vi "Tranzycja.vi"(7 "input":T2, 9 "Tranzycja":bool, 11 "Interlock":bool) -> (3 "Akcja":bool, 4 "output":T2)   [LabVIEW 2020]
uses:
  controls/Data.ctl
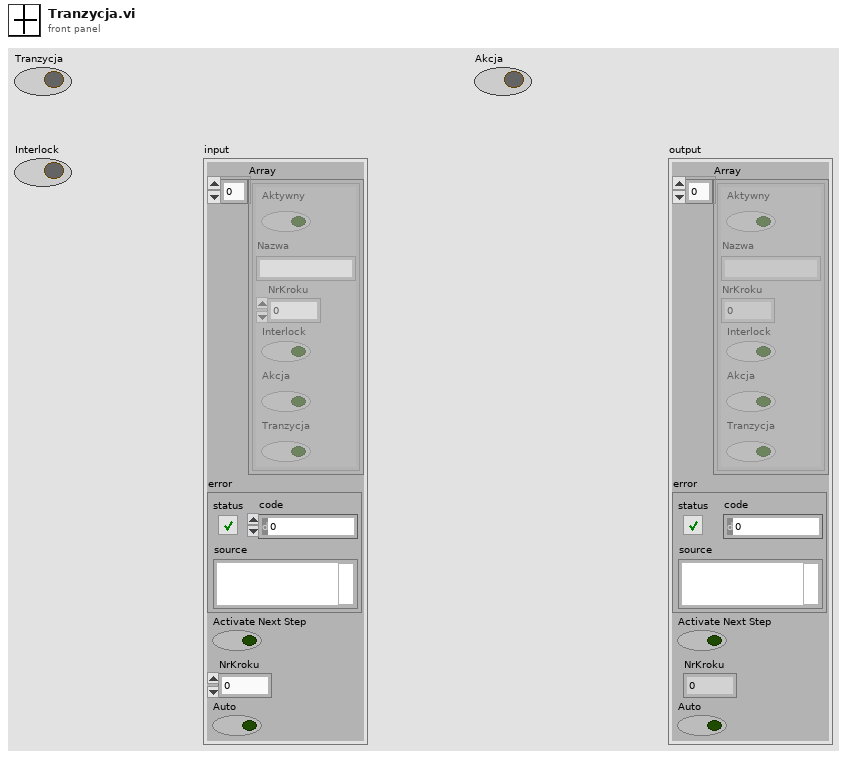
[diagram p1: front panel]
types:
  T1 = typedef "Data.ctl" = cluster{"Aktywny":bool, "Nazwa":string, "NrKroku":dbl, "Interlock":bool, "Akcja":bool, "Tranzycja":bool}
  T2 = cluster{"Array":T1[], "error":errorcluster, "Activate Next Step":bool, "NrKroku":dbl, "Auto":bool}
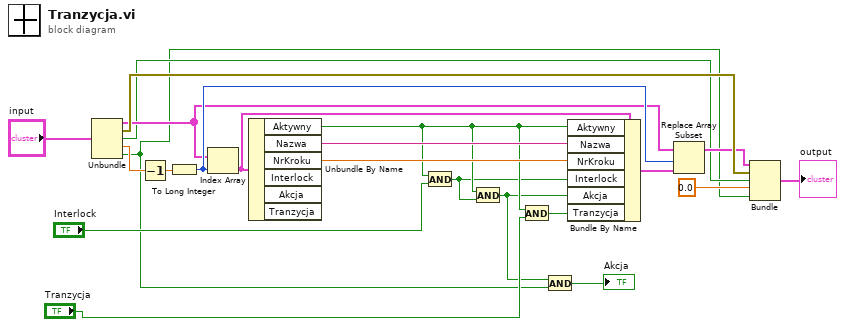
[diagram p0: block diagram]
diagram:
  n1 = Unbundle("input") -> ("Array"=w16:T1[], "error"=w21:errorcluster, "Activate Next Step"=w6:bool, "NrKroku"=w13:dbl, "Auto"=w1:bool)
  n2 = Decrement(x=w13) -> (x-1=w12:dbl)
  n3 = To Long Integer(number=w12) -> (32bit integer=w17:i32)
  n4 = Index Array(array=w16, index=w17) -> (element=w18:T1)
  n5 = Unbundle By Name(w18) -> ("Aktywny"=w5:bool, "Nazwa"=w14:string, "NrKroku"=w15:dbl)  [unwired: 3 out]
  n6 = And(x=w5, y="Interlock") -> (x .and. y?=w4:bool)
  n7 = And(x=w5, y=w4) -> (x .and. y?=w2:bool)
  n8 = And(x=w5, y="Tranzycja") -> (x .and. y?=w9:bool)
  n9 = And(x=w2, y=w1) -> (x .and. y?=→"Akcja":bool)
  n10 = Bundle By Name(cluster=w18, "Aktywny"=w5, "Nazwa"=w14, "NrKroku"=w15, "Interlock"=w4, "Akcja"=w2, "Tranzycja"=w9) -> (w19:T1)
  n11 = Replace Array Subset(array=w16, new element=w19, index=w17) -> (w20:T1[])
  n12 = Bundle("Array"=w20, "error"=w21, "Activate Next Step"=w6, "NrKroku"=0.0, "Auto"=w1) -> (→"output":T2)  [unwired: 1 in]
